vi "HDLC_byte_receive.vi"(10 "new_byte":u8) -> (1 "frame_size":u8, 2 "data_type":T1, 3 "frame":u8[](array[numeric]))   [LabVIEW 2018]
uses:
  data_frame_types/frame_data_type.ctl
  special_characters.ctl
  crc16_initial_val.ctl
panel:
  in  "local_data":T2={"frame_buffer"=[], "prev_was_escape"=FALSE, "frame_pos"=0, "checksum"=65535, "max_frame_size"=64} {"checksum" format="%x"}
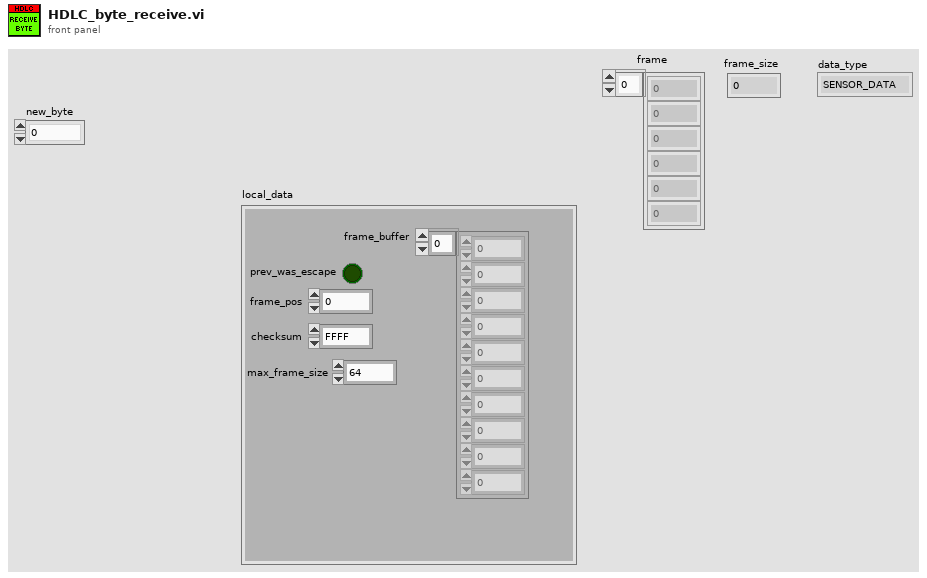
[diagram p1: front panel]
types:
  T1 = typedef "frame_data_type.ctl" = enum8{"SENSOR_DATA", "RND_MAX"}
  T2 = cluster{"frame_buffer":u8[], "prev_was_escape":bool, "frame_pos":u8, "checksum":u16, "max_frame_size":u8}
  T3 = typedef "special_characters.ctl" = u8
  T4 = typedef "crc16_initial_val.ctl" = u16
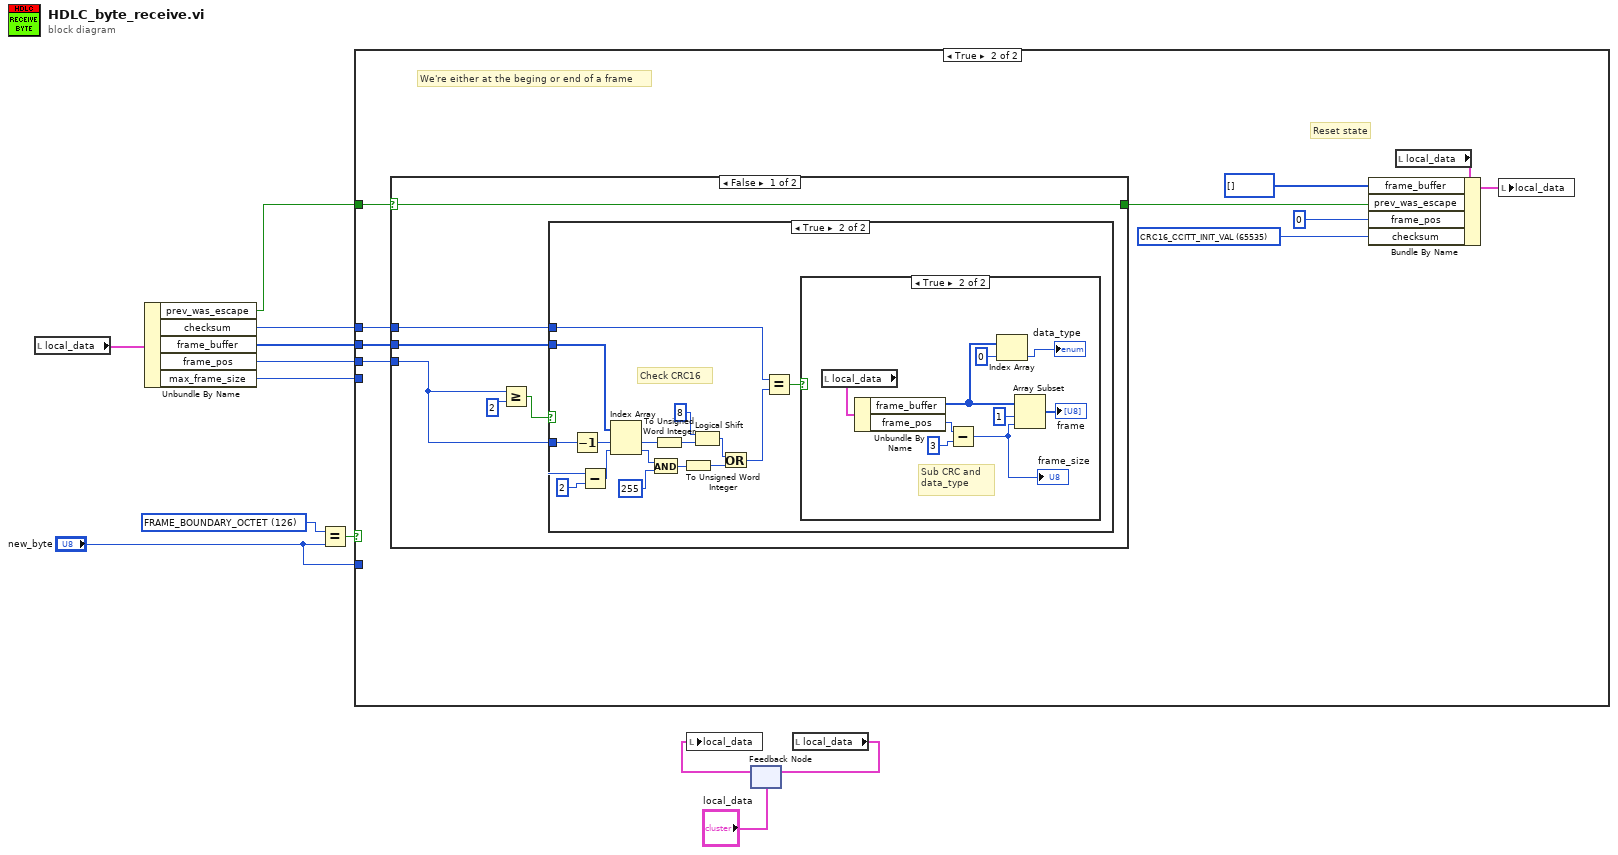
[diagram p0: block diagram]
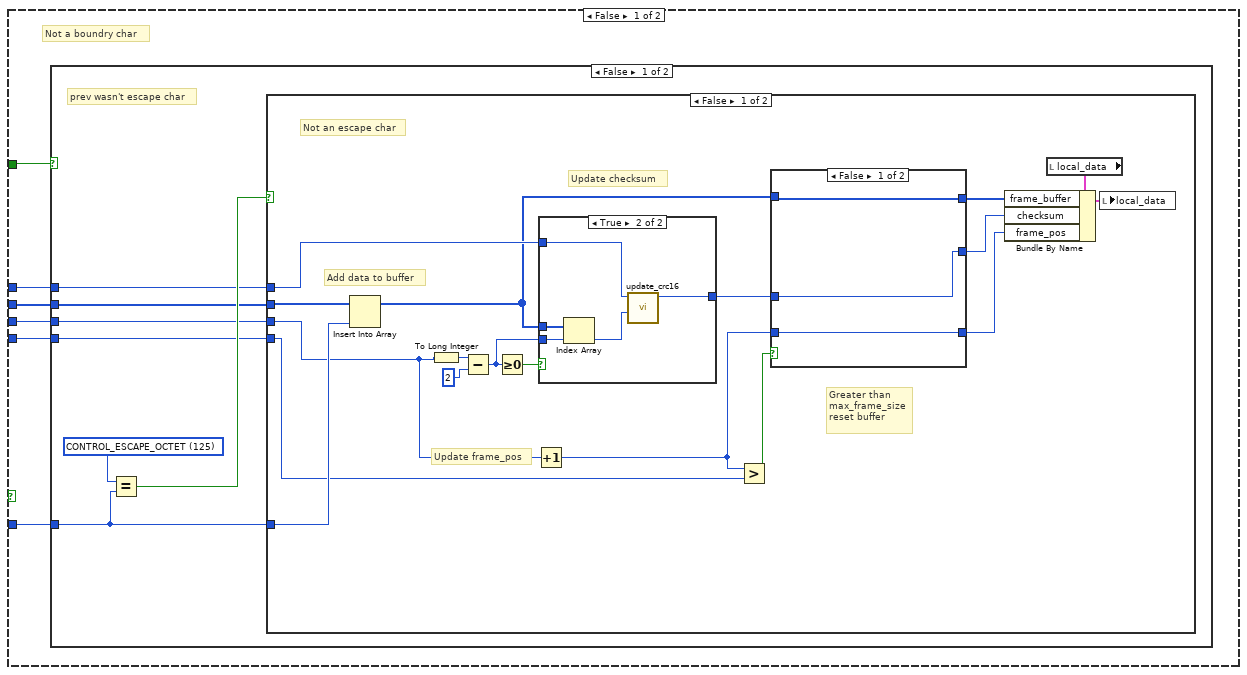
[diagram p2: hidden frame]
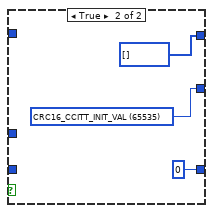
[diagram p3: hidden frame]
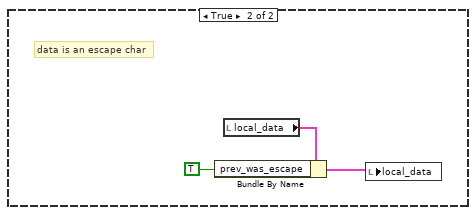
[diagram p5: hidden frame]
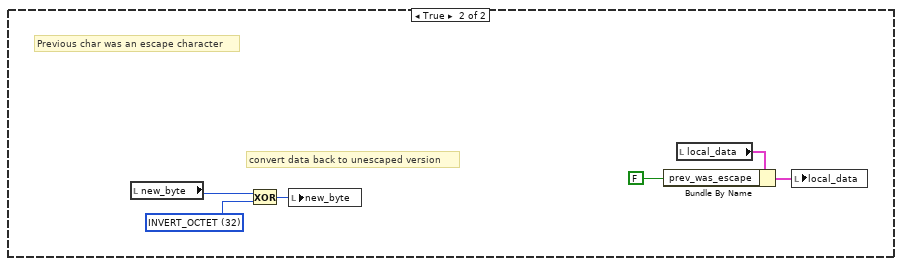
[diagram p6: hidden frame]
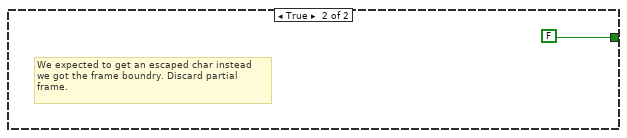
[diagram p9: hidden frame]
diagram:
  w12 = T3 126 items=["FRAME_BOUNDARY_OCTET"=126, "CONTROL_ESCAPE_OCTET"=125, "INVERT_OCTET"=32] ("Ring")
  n1 = local read "local_data"() -> (w10:T2)
  n2 = Unbundle By Name(w10) -> ("prev_was_escape"=w4:bool, "checksum"=w3:u16, "frame_buffer"=w6:u8[], "frame_pos"=w5:u8, "max_frame_size"=w1:u8)
  n3 = Equal?(x=w12, y="new_byte") -> (x = y?=w11:bool)
  n4 = case shown="True" w11 {
    tunnel: w6 -> [w16 w74]
    tunnel: w5 -> [w15 w73]
    tunnel: w4 -> [w18 w72]
    tunnel: w3 -> [w14 w71]
    tunnel: "new_byte" -> [w17 _]
    tunnel: w1 -> [w13 _]
    frame False {
      # "Not a boundry char"
      n5 = case shown="False" w18 {
        tunnel: w17 -> [w22 _]
        tunnel: w16 -> [w23 _]
        tunnel: w15 -> [w21 _]
        tunnel: w14 -> [w20 _]
        tunnel: w13 -> [w19 _]
        frame False {
          w25 = T3 125 items=["FRAME_BOUNDARY_OCTET"=126, "CONTROL_ESCAPE_OCTET"=125, "INVERT_OCTET"=32] ("Ring")
          # "prev wasn't escape char"
          n6 = Equal?(x=w25, y=w22) -> (x = y?=w24:bool)
          n7 = case shown="False" w24 {
            tunnel: w23 -> [w43 _]
            tunnel: w22 -> [w42 _]
            tunnel: w21 -> [w26 _]
            tunnel: w20 -> [w37 _]
            tunnel: w19 -> [w34 _]
            frame False {
              # "Greater than\nmax_frame_size\nreset buffer"
              # "Update frame_pos"
              # "Update checksum"
              # "Add data to buffer"
              # "Not an escape char"
              n8 = Insert Into Array(array=w43, new element=w42) -> (w28:u8[])  [unwired: 1 in]
              n9 = To Long Integer(number=w26) -> (32bit integer=w27:i32)
              n10 = Subtract(x=w27, y=2) -> (x-y=w36:i32)
              n11 = Greater Or Equal To 0?(x=w36) -> (x >= 0?=w38:bool)
              n12 = Increment(x=w26) -> (x+1=w33:u8)
              n13 = case shown="True" w38 {
                tunnel: w37 -> [w50 w53]
                tunnel: w28 -> [_ w55]
                tunnel: w36 -> [_ w54]
                tunnel: [w50 w51] -> w30
                frame False {
                }
                frame True {
                  n14 = Index Array(array=w55, index=w54) -> (element=w52:u8)
                  n15 = call "update_crc16.vi"("data"=w52, "crc"=w53) -> ("new_crc"=w51:u16)  [unwired: 9 in]
                }
              }
              n16 = Greater?(x=w33, y=w34) -> (0:w35:bool)
              n17 = case shown="False" w35 {
                tunnel: w33 -> [w46 _]
                tunnel: [w46 u8 0] -> w32
                tunnel: [w45 w48] -> w31
                tunnel: w30 -> [w45 _]
                tunnel: w28 -> [w44 _]
                tunnel: [w44 u8[] []] -> w29
                frame False {
                }
                frame True {
                  w48 = T4 65535 items=["CRC16_CCITT_INIT_VAL"=65535] ("CRC16")
                }
              }
              n18 = local read "local_data"() -> (w41:T2)
              n19 = Bundle By Name(cluster=w41, "frame_buffer"=w29, "checksum"=w31, "frame_pos"=w32) -> (w40:T2)
              n20 = local write "local_data"(w40) -> ()
            }
            frame True {
              # "data is an escape char"
              n21 = local read "local_data"() -> (w58:T2)
              n22 = Bundle By Name(cluster=w58, "prev_was_escape"=TRUE) -> (w57:T2)
              n23 = local write "local_data"(w57) -> ()
            }
          }
        }
        frame True {
          w63 = T3 32 items=["FRAME_BOUNDARY_OCTET"=126, "CONTROL_ESCAPE_OCTET"=125, "INVERT_OCTET"=32] ("Ring")
          # "convert data back to unescaped version"
          # "Previous char was an escape character"
          n24 = local read "new_byte"() -> (w64:u8)
          n25 = Exclusive Or(1:w63, 2:w64) -> (0:w62:T3)
          n26 = local write "new_byte"(w62) -> ()
          n27 = local read "local_data"() -> (w61:T2)
          n28 = Bundle By Name(cluster=w61, "prev_was_escape"=FALSE) -> (w60:T2)
          n29 = local write "local_data"(w60) -> ()
        }
      }
    }
    frame True {
      w68 = T4 65535 items=["CRC16_CCITT_INIT_VAL"=65535] ("CRC16")
      # "Reset state"
      # "We're either at the beging or end of a frame"
      n30 = case shown="False" w72 {
        selector: w72 -> [w80 _]
        tunnel: [w80 FALSE] -> w65
        tunnel: w74 -> [w78 _]
        tunnel: w73 -> [w77 _]
        tunnel: w71 -> [w75 _]
        frame False {
          n31 = Greater Or Equal?(x=w77, y=u8 2) -> (x >= y?=w76:bool)
          n32 = case shown="True" w76 {
            tunnel: w78 -> [_ w86]
            tunnel: w77 -> [_ w85]
            tunnel: w75 -> [_ w84]
            frame False {
            }
            frame True {
              # "Check CRC16"
              n33 = Decrement(x=w85) -> (x-1=w96:u8)
              n34 = Subtract(x=w85, y=u8 2) -> (x-y=w95:u8)
              n35 = Index Array(array=w86, index #1=w96, index #2=w95) -> (element #1=w82:u8, element #2=w81:u8)
              n36 = And(x=w81, y=u8 255) -> (x .and. y?=w88:u8)
              n37 = To Unsigned Word Integer(number=w82) -> (unsigned 16bit integer=w90:u16)
              n38 = To Unsigned Word Integer(number=w88) -> (unsigned 16bit integer=w87:u16)
              n39 = Logical Shift(y=i16 8, x=w90) -> (x << y=w92:u16)
              n40 = Or(x=w92, y=w87) -> (x .or. y?=w91:u16)
              n41 = Equal?(x=w84, y=w91) -> (x = y?=w83:bool)
              n42 = case shown="True" w83 {
                frame False {
                }
                frame True {
                  # "Sub CRC and \ndata_type"
                  n43 = local read "local_data"() -> (w105:T2)
                  n44 = Unbundle By Name(w105) -> ("frame_buffer"=w99:u8[], "frame_pos"=w104:u8)
                  n45 = Subtract(x=w104, y=u8 3) -> (x-y=w101:u8)
                  "frame_size" <- w101
                  n46 = Index Array(array=w99, index=0) -> (element=→"data_type":u8)
                  n47 = Array Subset(array=w99, index=1, length=w101) -> (→"frame":u8[])
                }
              }
            }
          }
        }
        frame True {
          # "We expected to get an escaped char instead \nwe got the frame boundry. Discard partial\nframe."
        }
      }
      n48 = local read "local_data"() -> (w70:T2)
      n49 = Bundle By Name(cluster=w70, "frame_buffer"=u8[] [], "prev_was_escape"=w65, "frame_pos"=u8 0, "checksum"=w68) -> (w69:T2)
      n50 = local write "local_data"(w69) -> ()
    }
  }
  n51 = feedback #1("local_data") -> (w7:T2)
  n52 = local write "local_data"(w7) -> ()
  n53 = local read "local_data"() -> (w8:T2)
  n54 = feedback-in #1(w8) -> ()
